vi "Test Example Polymorphic 1.vi"() -> ()   [LabVIEW 2014]
panel:
  out "VI Name":string
  in  "vi path":path=path "C:/Users/lubo/Documents/LabView/LabVIEW-Universal-Transcriptor/Test/Examples For Parsing/Example Polymorphic 1.vi"
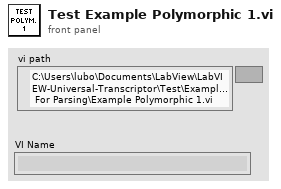
[diagram p1: front panel]
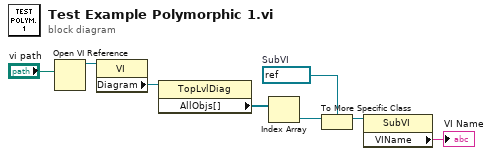
[diagram p0: block diagram]
diagram:
  w5 = refnum<vi> refnum  # SubVI
  n1 = Open VI Reference(vi path="vi path") -> (vi reference=w7:refnum<vi>)  [unwired: 5 in, 1 out]
  n2 = property class="VI"(reference=w7) -> ("Diagram"=w6:refnum<vi>)  [unwired: 1 in, 2 out]
  n3 = property class="TopLvlDiag"(reference=w6) -> ("AllObjs[]"=w4:refnum<vi>[])  [unwired: 1 in, 2 out]
  n4 = Index Array(array=w4) -> (element=w3:refnum<vi>)  [unwired: 1 in]
  n5 = To More Specific Class(target class=w5, reference=w3) -> (specific class reference=w1:refnum<vi>)  [unwired: 1 in, 1 out]
  n6 = property class="SubVI"(reference=w1) -> ("VIName"=→"VI Name":string)  [unwired: 1 in, 2 out]
